vi "Software Principal.vi"() -> ()   [LabVIEW 2017]
uses:
  <vilib>/DAQmx/read.llb/DAQmx Read (Analog 1D Wfm NChan NSamp).vi
  <vilib>/DAQmx/read.llb/DAQmx Read (Analog DBL 1Chan 1Samp).vi
  <vilib>/DAQmx/create/channels.llb/DAQmx Create Channel (AI-Strain-Strain Gage).vi
  <vilib>/DAQmx/configure/timing.llb/DAQmx Timing (Sample Clock).vi
  <vilib>/DAQmx/calibration/calibrationInfo.llb/DAQmx Perform Shunt Calibration Ex (Strain).vi
  <vilib>/DAQmx/create/channels.llb/DAQmx Create Channel (AI-Temperature-Thermocouple).vi
  <vilib>/express/express shared/transition.llb/Dynamic To Waveform Array.vi
  <vilib>/express/express signal manip/GetorSetDDTAttributes/Set DDT Attributes/SetT0.vi
  <vilib>/express/express shared/transition.llb/Waveform Array To Dynamic.vi
  <vilib>/DAQmx/miscellaneous.llb/DAQmx Fill In Error Info.vi
  <vilib>/express/express signal manip/GetorSetDDTAttributes/Set DDT Attributes/Set DDT Properties.xnode
panel:
  out "Tempo corrido (s)":dbl
  in  "?":T1(tab)=enum."SETTINGS OF THE TEST "
  out "Voltage applied in the valve":dbl(knob) scale=0.0..10.0 scale format="%#_gV"
  out "Voltage applied in the voltage source":dbl(knob) scale=0.0..10.0 scale format="%#_gV"
  out "Deformation":waveform(dbl)[](graph)
  out "VALVE ON":bool
  out "VOLTAGE SOURCE ON":bool
  out "Temperature":dbl(graph)
  out "Temperature (°C)":dbl format="%#_g °C"
  in  "?":bool
  out "Number of cycles":dbl
  in  "MINIMUM TEMPERATURE OF THE TEST":dbl
  in  "MAXIMUM TEMPERATURE OF THE TEST":dbl
  in  "NUMBER OF CYCLES":dbl
  in  "DIRECTORY TO STORE THE DATA":path=path "C:/Users/Luis/Desktop/RIQUELME/SOFTWARE PRINCIPAL/REGISTRODEDADOS/DadosEnsaioFadiga.tdms" caption="Filename"
  in  "?":T2(tab)
  in  "INFORMA钦ES DA PONTE":T3={"TIPO DE PONTE"=10183, "RESISTÊNCIA DO FIO"=0.0, "TENSÃO INICIAL DA PONTE"=0.0, "TIPO DE EXCITA敲O DA PONTE"=10200, "TENSÃO DE EXCITAÇÃO"=2.5} {"TIPO DE PONTE" items=["Full Bridge I"=10183, "Full Bridge II"=10184, "Full Bridge III"=10185, "Half Bridge I"=10188, "Half Bridge II"=10189, "Quarter Bridge I"=10271, "Quarter Bridge II"=10272]; "TIPO DE EXCITA敲O DA PONTE" items=["Internal"=10200, "External"=10167, "None"=10230]}
  in  "INFORMAÇÕES DO EXTENSÔMETRO":T4={"GAGE FACTOR"=2.0, "RESISTÊNCIA DO EXTENSÔMETRO"=350.0, "COEFICIENTE DE POISSON"=0.3}
  in  "HABILITA敲O DE DESLOCAMENTO NULO":bool
  in  "CALIBRA敲O DE SHUNT":bool
  # "Diagrama de conexão Quarter-Bridge para a aquisição de dados de cada extensômetro"
  # "Especificação de cada pino NI 9949"
  # "Diagrama de Conexão para a Aquisição de Dados do Termopar"
  # "Diagrama de Conexão para Controle da Fonte via tensão externa ( 0-10V)"
  # "Diagrama de Conexão para operar a fonte Manualmente - as conexões em pontilhado não precisam ser feitas"
  # "Diagrama de Conexão para o Controle da Válvula via Tensão Externa"
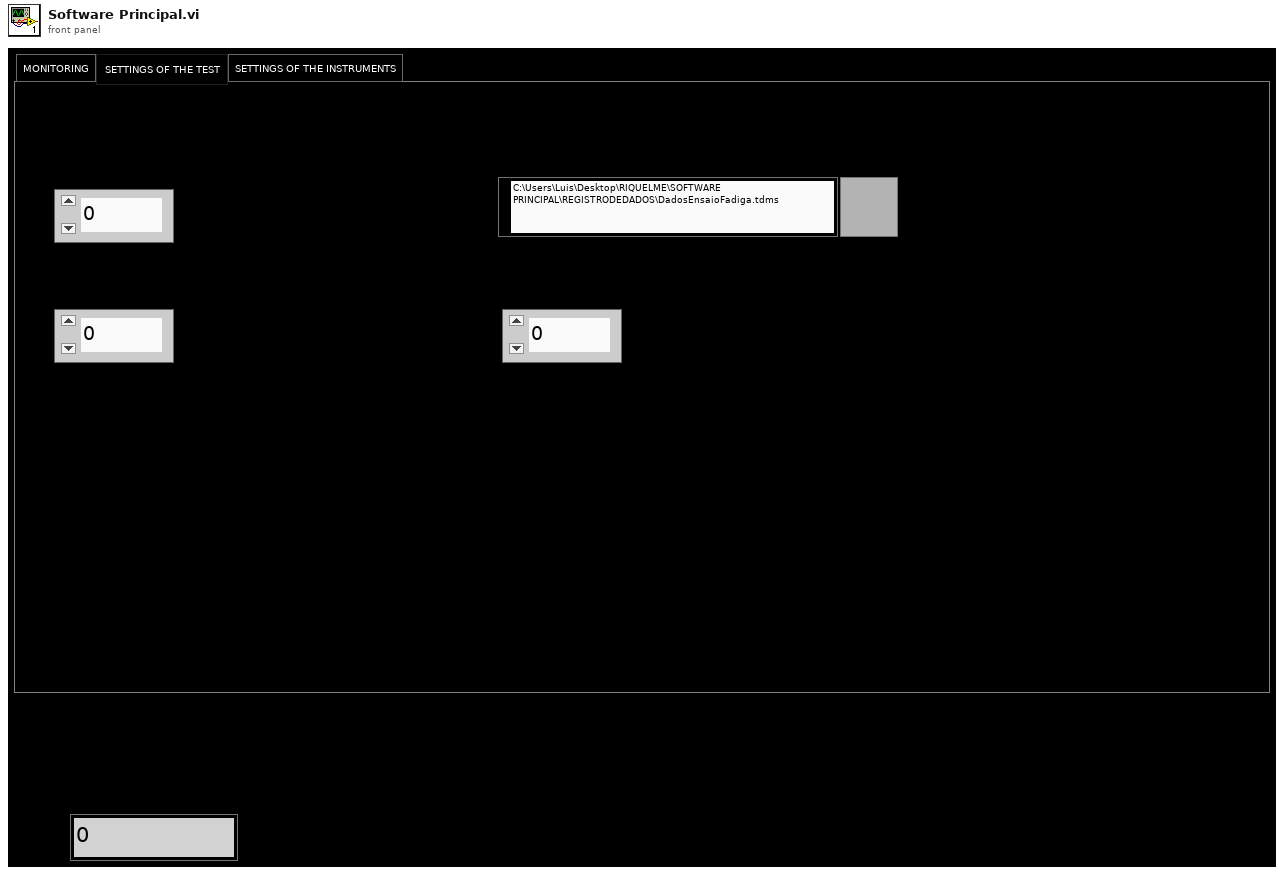
[diagram p1: front panel]
types:
  T1 = enum32{"MONITORING", "SETTINGS OF THE TEST ", "SETTINGS OF THE INSTRUMENTS"}
  T2 = enum32{"EXTENSÔMETROS", "TERMOPAR", "FONTE DE TENSÃO", "VÁLVULA"}
  T3 = cluster{"TIPO DE PONTE":i32, "RESISTÊNCIA DO FIO":dbl, "TENSÃO INICIAL DA PONTE":dbl, "TIPO DE EXCITA敲O DA PONTE":i32, "TENSÃO DE EXCITAÇÃO":dbl}
  T4 = cluster{"GAGE FACTOR":dbl, "RESISTÊNCIA DO EXTENSÔMETRO":dbl, "COEFICIENTE DE POISSON":dbl}
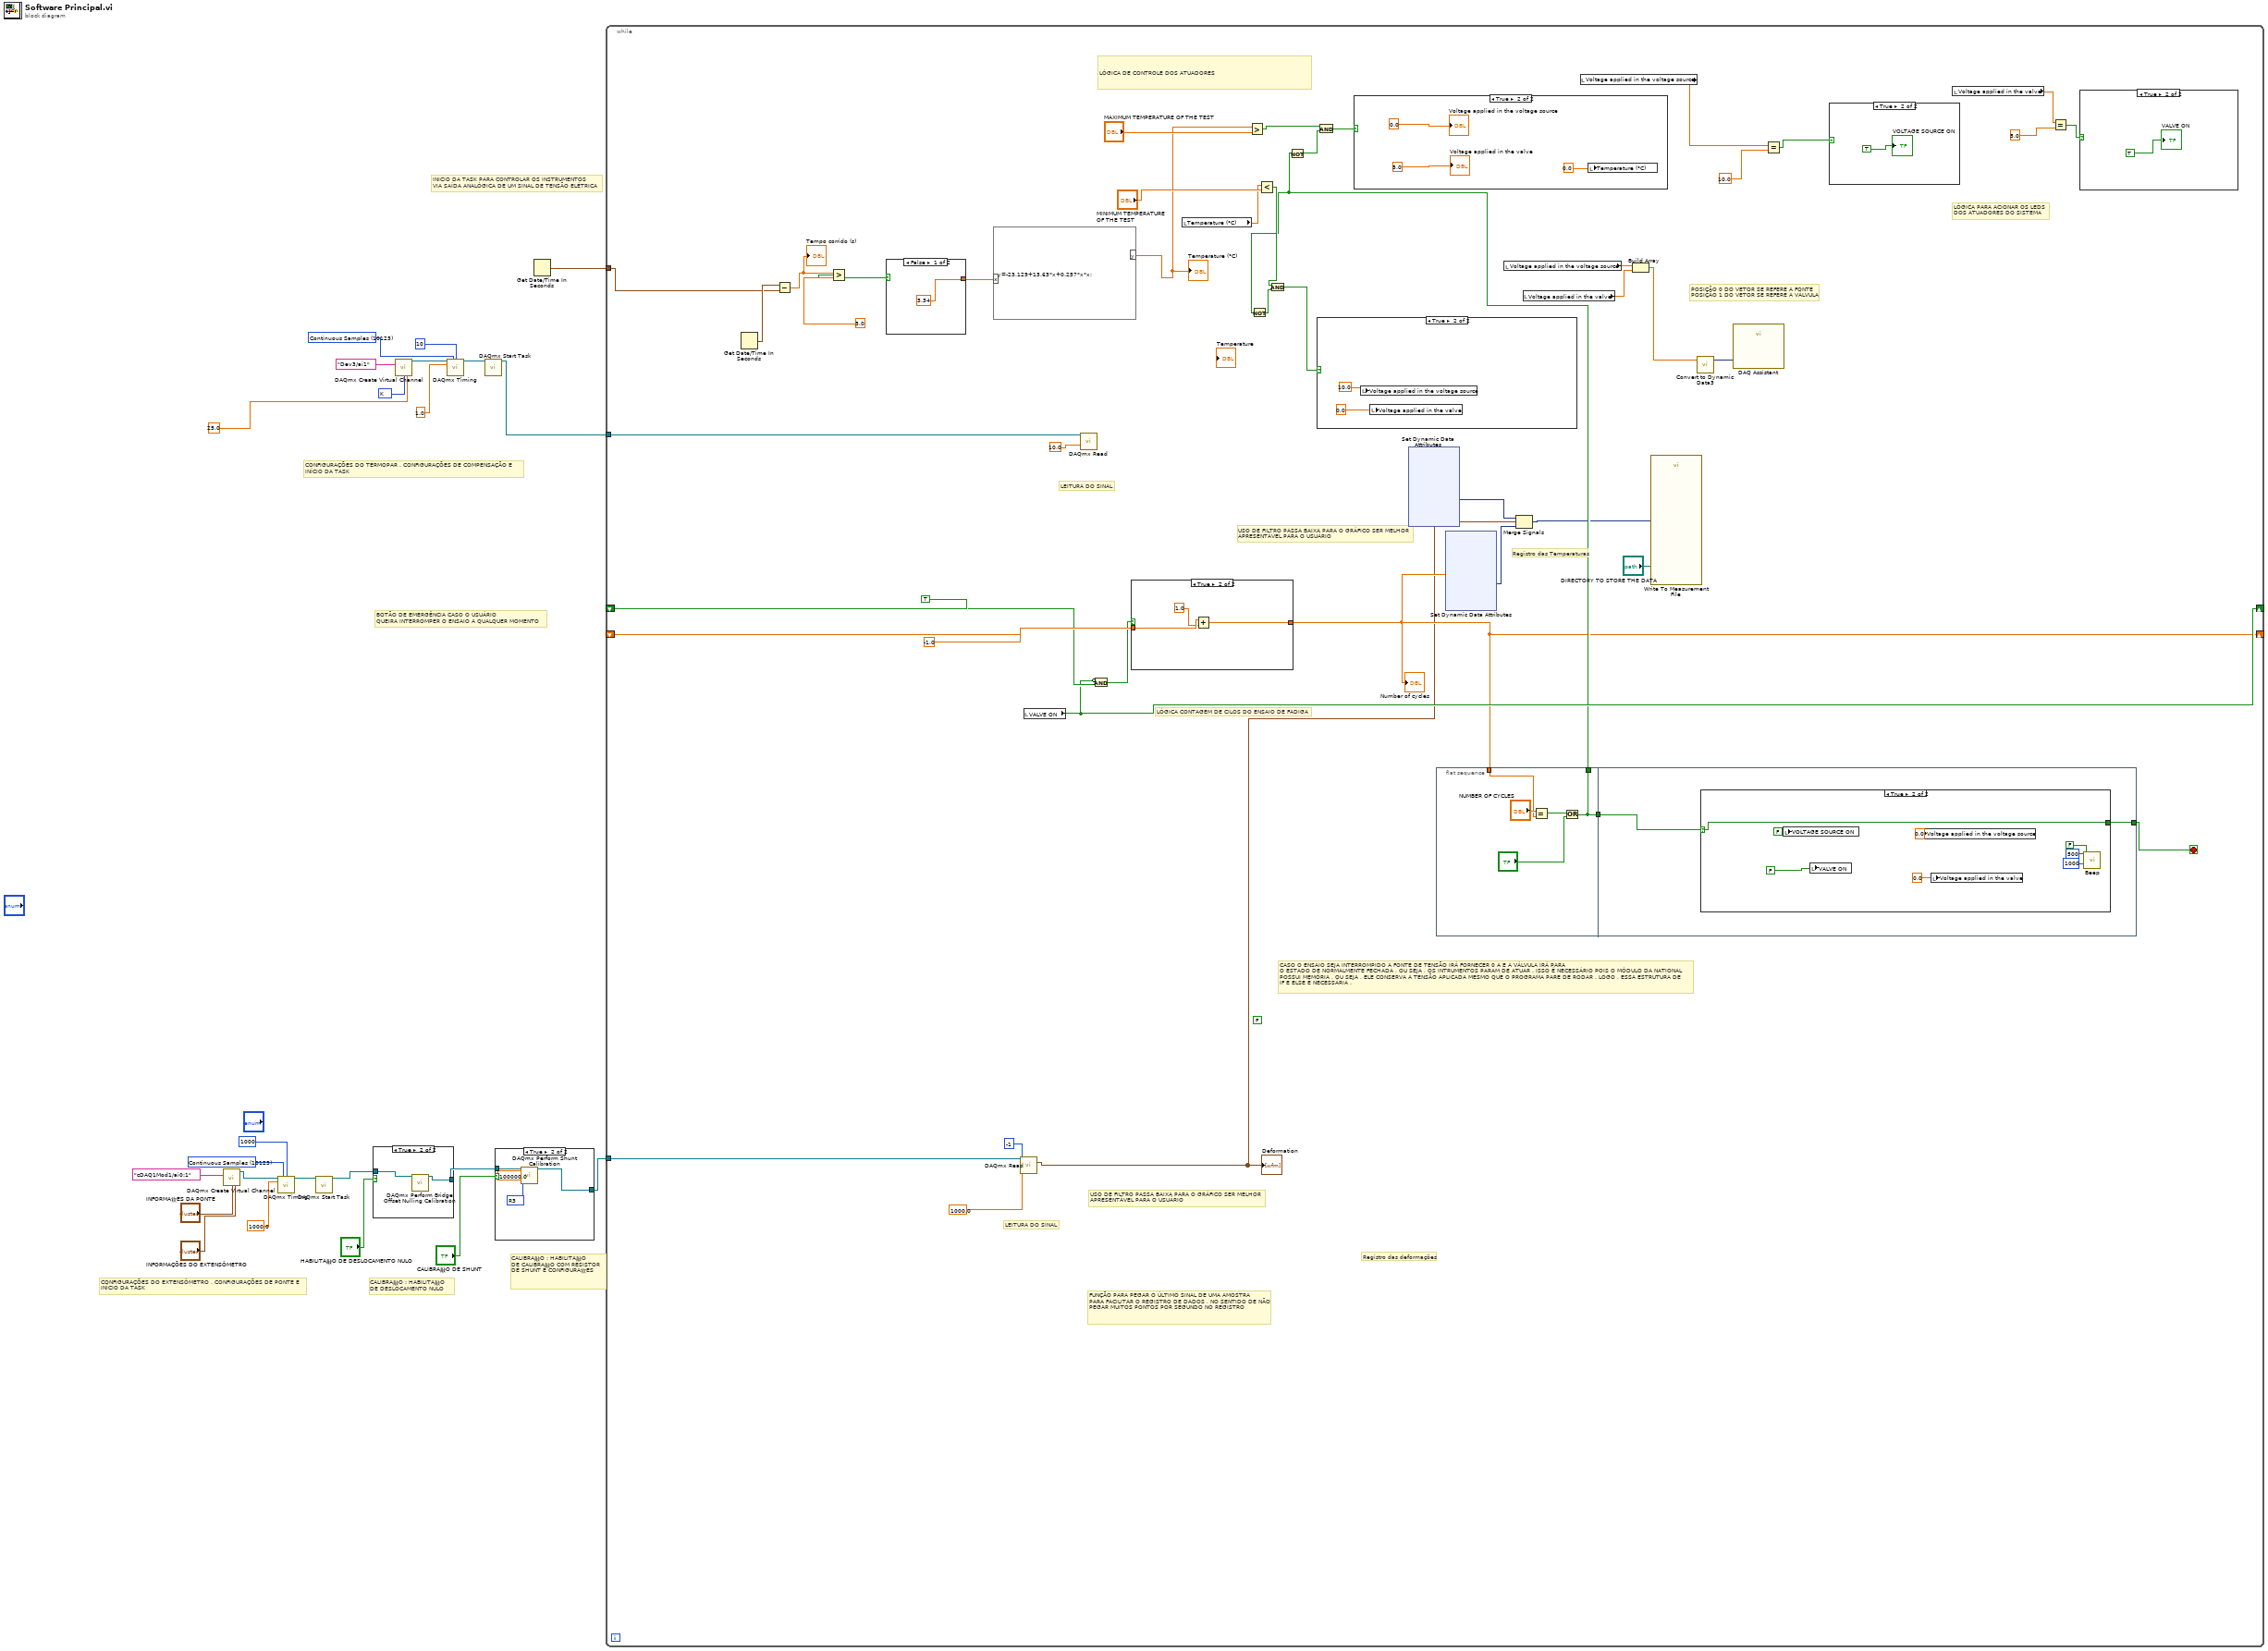
[diagram p0: block diagram]
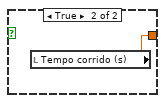
[diagram p4: hidden frame]
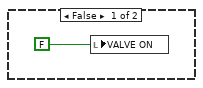
[diagram p7: hidden frame]
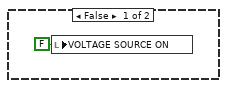
[diagram p8: hidden frame]
diagram:
  w19 = 10073 items=["J"=10072, "K"=10073, "N"=10077, "R"=10082, "S"=10085, "T"=10086, "B"=10047, "E"=10055] ("TIPO DO TERMOPAR")
  w10 = 10123 items=["Finite Samples"=10178, "Continuous Samples"=10123, "Hardware Timed Single Point"=12522] ("sample mode")
  w24 = 10123 items=["Finite Samples"=10178, "Continuous Samples"=10123, "Hardware Timed Single Point"=12522] ("sample mode")
  # "CALIBRA敲O : HABILITA敲O\nDE CALIBRA敲O COM RESISTOR\nDE SHUNT E CONFIGURA钦ES"
  # "CALIBRA敲O : HABILITA敲O\nDE DESLOCAMENTO NULO"
  # "CONFIGURAÇÕES DO EXTENSÔMETRO , CONFIGURAÇÕES DE PONTE E  \nINÍCIO DA TASK"
  # "BOTÃO DE EMERGÊNCIA CASO O USUÁRIO\nQUEIRA INTERROMPER O ENSAIO A QUALQUER MOMENTO"
  # "INICIO DA TASK PARA CONTROLAR OS INSTRUMENTOS\nVIA SAÍDA ANALÓGICA DE UM SINAL DE TENSÃO ELÉTRICA"
  # "CONFIGURAÇÕES DO TERMOPAR , CONFIGURAÇÕES DE COMPENSAÇÃO E  \nINÍCIO DA TASK"
  n1 = call-poly <vilib>:"DAQmx Create Virtual Channel.vi"("physical channels"=tag "cDAQ1Mod1/ai0:1", "bridge information"="INFORMA钦ES DA PONTE", "strain gage information"="INFORMAÇÕES DO EXTENSÔMETRO") -> ("task out"=w11:refnum<k21>)  [unwired: 11 in, 1 out]
  n2 = call-poly <vilib>:"DAQmx Timing.vi"("task/channels in"=w11, "sample mode"=w10, "samples per channel"=1000, "rate"=1000.0) -> ("task out"=w8:refnum<k21>)  [unwired: 10 in, 1 out]
  n3 = call <vilib>:"DAQmx Start Task.vi"("task/channels in"=w8) -> ("task out"=w3:refnum<k21>)  [unwired: 13 in, 1 out]
  n4 = case shown="True" "HABILITA敲O DE DESLOCAMENTO NULO" {
    tunnel: [w26 w28] -> w5
    tunnel: w3 -> [w26 w27]
    frame False {
    }
    frame True {
      n5 = call <vilib>:"DAQmx Perform Bridge Offset Nulling Calibration.vi"("task/channels in"=w27) -> ("task out"=w28:refnum<k21>)  [unwired: 13 in, 1 out]
    }
  }
  n6 = call-poly <vilib>:"DAQmx Create Virtual Channel.vi"("physical channels"=tag "Dev3/ai1", "thermocouple type"=w19, "cjc value"=25.0 ("FATOR DE COMPENSA敲O CJC")) -> ("task out"=w25:refnum<k21>)  [unwired: 11 in, 1 out]
  n7 = call-poly <vilib>:"DAQmx Timing.vi"("task/channels in"=w25, "sample mode"=w24, "samples per channel"=10, "rate"=1.0) -> ("task out"=w21:refnum<k21>)  [unwired: 10 in, 1 out]
  n8 = call <vilib>:"DAQmx Start Task.vi"("task/channels in"=w21) -> ("task out"=w17:refnum<k21>)  [unwired: 13 in, 1 out]
  n9 = case shown="True" "CALIBRA敲O DE SHUNT" {
    tunnel: w5 -> [w29 w33]
    tunnel: [w29 w30] -> w2
    frame False {
    }
    frame True {
      w31 = 12467 items=["R1"=12465, "R2"=12466, "R3"=12467, "R4"=14813] ("shunt element location")
      n10 = call-poly <vilib>:"DAQmx Perform Shunt Calibration.vi"("task/channels in"=w33, "shunt resistance"=100000.0, "shunt element location"=w31) -> ("task out"=w30:refnum<k21>)  [unwired: 11 in, 1 out]
    }
  }
  n11 = Get Date/Time In Seconds() -> (seconds since 1Jan1904=w1:timestamp)
  n12 = while {
    tunnel: w17 -> [w64]
    shift-right: [w60] -> _
    shift-left: TRUE -> [w62]
    shift-right: [w49] -> _
    shift-left: -1.0 ("y") -> [w63]
    tunnel: w2 -> [w45]
    tunnel: w1 -> [w36]
    stop <- w58 stop-if-true
    (unwired) FALSE
    # "LEITURA DO SINAL"
    # "FUNÇÃO PARA PEGAR O ÚLTIMO SINAL DE UMA AMOSTRA\nPARA FACILITAR O REGISTRO DE DADOS , NO SENTIDO DE NÃO\nPEGAR MUITOS PONTOS POR SEGUNDO NO REGISTRO"
    # "USO DE FILTRO PASSA BAIXA PARA O GRÁFICO SER MELHOR\nAPRESENTÁVEL PARA O USUÁRIO"
    # "Registro das deformações"
    # "LÓGICA CONTAGEM DE CILOS DO ENSAIO DE FADIGA"
    # "CASO O ENSAIO SEJA INTERROMPIDO A FONTE DE TENSÃO IRÁ FORNECER 0 A E A VÁLVULA IRÁ PARA\nO ESTADO DE NORMALMENTE FECHADA , OU SEJA , OS INTRUMENTOS PARAM DE ATUAR . ISSO É NECESSÁRIO POIS O MÓDULO DA NATIONAL \nPOSSUI MEMÓRIA , OU SEJA , ELE CONSERVA A TENSÃO APLICADA MESMO QUE O PROGRAMA PARE DE RODAR . LOGO , ESSA ESTRUTURA DE \nIF E ELSE É NECESSÁRIA ."
    # "LÓGICA PARA ACIONAR OS LEDS\nDOS ATUADORES DO SISTEMA"
    # "POSIÇÃO 0 DO VETOR SE REFERE A FONTE\nPOSIÇÃO 1 DO VETOR SE REFERE A VÁLVULA"
    # "LEITURA DO SINAL"
    # "Registro das Temperaturas"
    # "USO DE FILTRO PASSA BAIXA PARA O GRÁFICO SER MELHOR\nAPRESENTÁVEL PARA O USUÁRIO"
    # "LÓGICA DE CONTROLE DOS ATUADORES"
    n13 = Get Date/Time In Seconds() -> (seconds since 1Jan1904=w41:timestamp)
    n14 = Subtract(x=w41, y=w36) -> (x-y=w38:dbl)
    "Tempo corrido (s)" <- w38
    n15 = Greater?(x=w38, y=3.0) -> (0:w39:bool)
    n16 = case shown="False" w39 {
      tunnel: [3.34 ("y") w79] -> w37
      frame False {
      }
      frame True {
        n17 = local read "Tempo corrido (s)"() -> (w79:dbl)
      }
    }
    n18 = formula code="y=-23.129+13.63*x+0.257*x*x;"("x"=w37) -> ("y"=w35:dbl)
    "Temperature (°C)" <- w35
    n19 = call-poly <vilib>:"DAQmx Read.vi"("task/channels in"=w45, "number of samples per channel"=-1, "timeout"=1000.0) -> ("data"=w42:waveform(dbl)[])  [unwired: 10 in, 2 out]
    "Deformation" <- w42
    n20 = local read "VALVE ON"() -> (w60:bool)
    n21 = call-poly <vilib>:"DAQmx Read.vi"("task/channels in"=w64, "timeout"=10.0) -> ()  [unwired: 11 in, 3 out]
    n22 = Compound Arithmetic op=AND(invert w60, w62) -> (w61:bool)
    n23 = case shown="True" w61 {
      tunnel: w63 -> [w124 w127]
      tunnel: [w124 w125] -> w49
      frame False {
      }
      frame True {
        n24 = Add(x=w127, y=1.0) -> (x+y=w125:dbl)
      }
    }
    "Number of cycles" <- w49
    n25 = local read "Temperature (°C)"() -> (w34:dbl)
    n26 = Greater?(x=w35, y="MAXIMUM TEMPERATURE OF THE TEST") -> (0:w57:bool)
    n27 = Not(x=w51) -> (.not. x?=w52:bool)
    n28 = Less?(x=w34, y="MINIMUM TEMPERATURE OF THE TEST") -> (x < y?=w53:bool)
    n29 = And(x=w53, y=w52) -> (x .and. y?=w54:bool)
    n30 = Not(x=w51) -> (.not. x?=w55:bool)
    n31 = case shown="True" w54 {
      frame False {
      }
      frame True {
        n32 = local write "Voltage applied in the voltage source"(10.0 ("TENSÃO APLICADA NA FONTE")) -> ()
        n33 = local write "Voltage applied in the valve"(0.0 ("TENSÃO APLICADA NA VÁLVULA")) -> ()
      }
    }
    n34 = And(x=w57, y=w55) -> (x .and. y?=w56:bool)
    n35 = case shown="True" w56 {
      frame False {
      }
      frame True {
        n36 = local write "Temperature (°C)"(0.0 ("Temperatura 2")) -> ()
        "Voltage applied in the voltage source" <- 0.0 ("TENSÃO APLICADA NA FONTE")
        "Voltage applied in the valve" <- 5.0 ("TENSÃO APLICADA NA VÁLVULA")
      }
    }
    n37 = xnode "Set Dynamic Data Attributes"() -> ("Signals Out"=w50:dynamicdata)  [unwired: 4 in, 1 out]
    n38 = flat-sequence {
      tunnel: w49 -> [w111]
      tunnel: [w108] -> w59
      tunnel: [w108] -> w51
      tunnel: w59 -> [w114]
      tunnel: [w113] -> w58
      frame #0 {
        n39 = Equal?(x="NUMBER OF CYCLES", y=w111) -> (x = y?=w110:bool)
        n40 = Or(x=w110, y="?") -> (x .or. y?=w108:bool)
      }
      frame #1 {
        n41 = case shown="True" w114 {
          selector: w114 -> [w115 w119]
          tunnel: [w115 w119] -> w113
          frame False {
          }
          frame True {
            n42 = local write "VOLTAGE SOURCE ON"(FALSE ("FONTE ATUANDO")) -> ()
            n43 = local write "VALVE ON"(FALSE ("VÁLVULA ATUANDO")) -> ()
            n44 = local write "Voltage applied in the voltage source"(0.0 ("TENSÃO APLICADA NA FONTE")) -> ()
            n45 = local write "Voltage applied in the valve"(0.0 ("TENSÃO APLICADA NA VÁLVULA")) -> ()
            n46 = call <vilib>:"Beep.vi"("use system alert? (T)"=FALSE, "duration (msec)"=u32 1000, "frequency (Hz)"=u32 500) -> ()  [unwired: 9 in]
          }
        }
      }
    }
    n47 = xnode "Set Dynamic Data Attributes"("Signals In"=w49) -> ("Signals Out"=w47:dynamicdata)  [unwired: 3 in, 1 out]
    n48 = local read "Voltage applied in the voltage source"() -> (w74:dbl)
    n49 = Merge Signals(w50, w42, w47) -> (w48:dynamicdata)
    n50 = local read "Voltage applied in the valve"() -> (w73:dbl)
    n51 = local read "Voltage applied in the voltage source"() -> (w72:dbl)
    n52 = Build Array(w74, w73) -> (w66:dbl[])
    n53 = call "Write To Measurement File"("Signals"=w48, "Filename"="DIRECTORY TO STORE THE DATA") -> ()  [unwired: 15 in, 3 out]
    n54 = call "Convert to Dynamic Data3"("Array"=w66) -> ("Dynamic Data Type"=w65:dynamicdata)  [unwired: 3 in]
    n55 = call "DAQ Assistant"("data"=w65) -> ()  [unwired: 17 in, 2 out]
    n56 = Equal?(x=w72, y=10.0) -> (x = y?=w70:bool)
    n57 = case shown="True" w70 {
      frame False {
        n58 = local write "VOLTAGE SOURCE ON"(FALSE ("FONTE ATUANDO")) -> ()
      }
      frame True {
        "VOLTAGE SOURCE ON" <- TRUE ("FONTE ATUANDO")
      }
    }
    n59 = local read "Voltage applied in the valve"() -> (w69:dbl)
    n60 = Equal?(x=w69, y=5.0) -> (x = y?=w67:bool)
    n61 = case shown="True" w67 {
      frame False {
        n62 = local write "VALVE ON"(FALSE ("VÁLVULA ATUANDO")) -> ()
      }
      frame True {
        "VALVE ON" <- TRUE ("VÁLVULA ATUANDO")
      }
    }
  }
